vi "Calculate_(11)_Local_Cost_F()-1.vi"(4 "[IN] Dot matrix with statuses \nfor potentially moving dots":i16[][](array[numeric]), 5 "[IN] Still connected\ntracks in group":T1, 6 "[IN] Potentially\nMoving (X,Y)":dbl[][](array[numeric]), 7 "[IN] Subtracks":T2(array[cluster]), 8 "error IN":errorcluster, 9 "[IN] Areas particles\nPrimary Detected":dbl[][](array[numeric]), 10 "[IN] Primary \n(X,Y) Detected":dbl[][](array[numeric]), 11 "[IN] Cost function":i8[](array[numeric])) -> (0 "error OUT":errorcluster, 3 "[OUT] Cost function":i8[](array[numeric]))   [LabVIEW 2013]
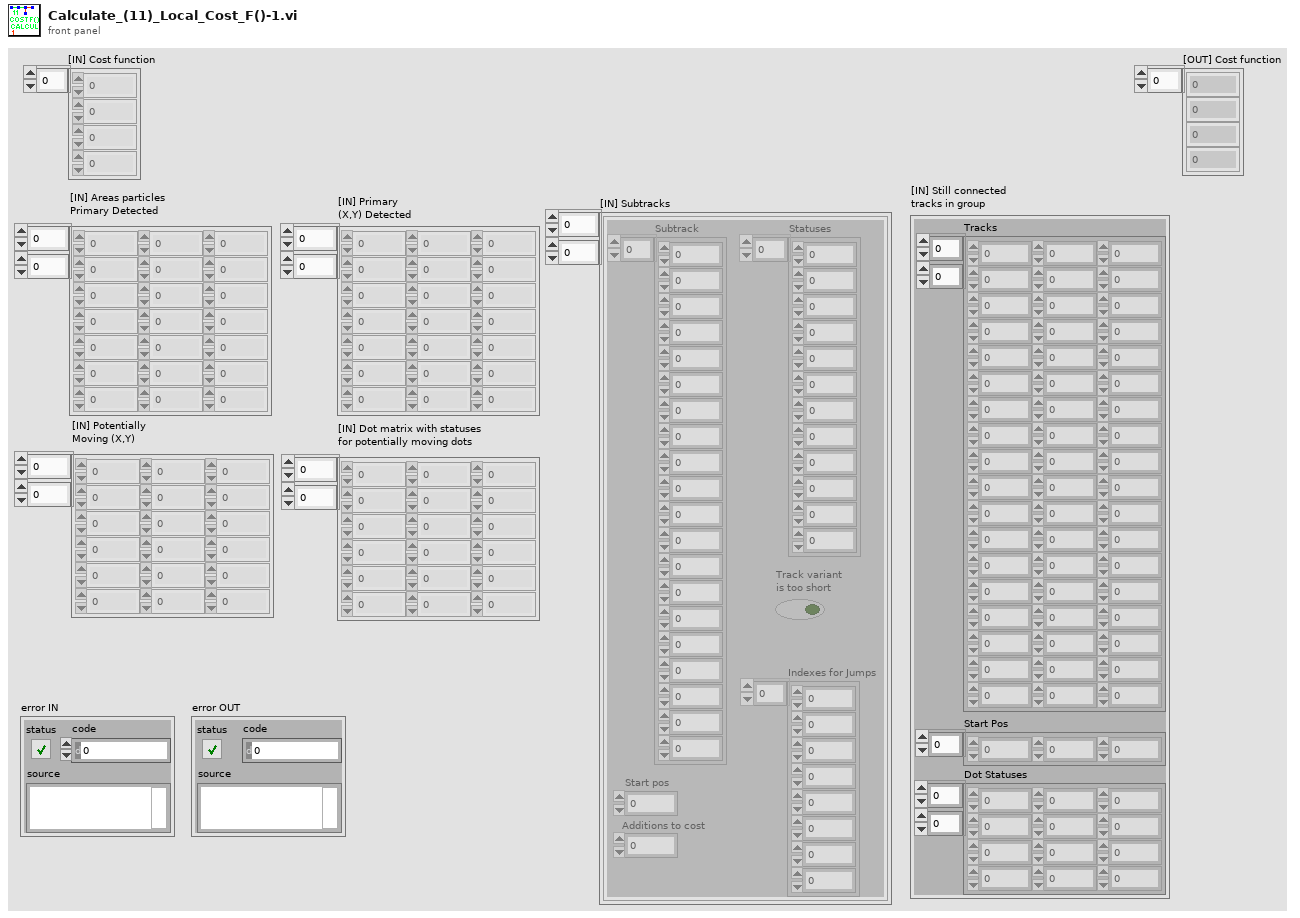
[diagram p1: front panel]
types:
  T1 = cluster{"Tracks":dbl[][], "Start Pos":i32[], "Dot Statuses":i16[][]}
  T2 = cluster{"Subtrack":dbl[], "Statuses":i16[], "Start pos":i32, "Additions to cost":i32, "Track variant \nis too short":bool, "Indexes for Jumps":i32[]}[][]
  T3 = cluster{"Subtrack":dbl[], "Statuses":i16[], "Start pos":i32, "Additions to cost":i32, "Track variant \nis too short":bool, "Indexes for Jumps":i32[]}[]
  T4 = cluster{"Subtrack":dbl[], "Statuses":i16[], "Start pos":i32, "Additions to cost":i32, "Track variant \nis too short":bool, "Indexes for Jumps":i32[]}
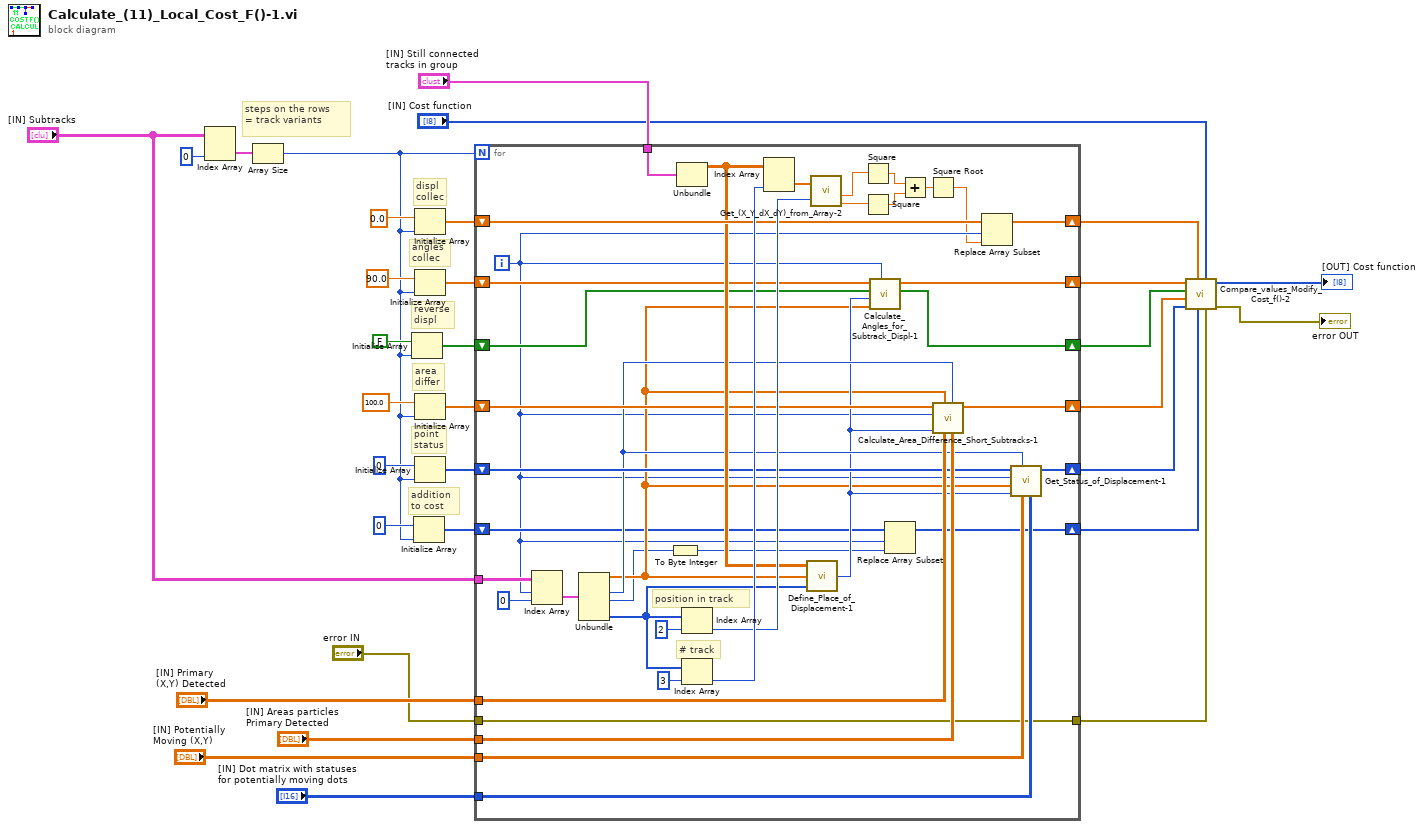
[diagram p0: block diagram]
diagram:
  # "steps on the rows\n= track variants"
  # "addition \nto cost"
  # "point\nstatus"
  # "area \ndiffer"
  # "reverse \ndispl"
  # "angles \ncollec"
  # "displ \ncollec"
  n1 = Index Array(array="[IN] Subtracks", index (col)=0 ("disabled index (col)")) -> (element=w18:T3)  [unwired: 1 in]
  n2 = Array Size(array=w18) -> (size(s)=w17:i32)
  n3 = Initialize Array(FALSE, w17) -> (w27:bool[])
  n4 = Initialize Array(i8 0, w17) -> (w21:i8[])
  n5 = Initialize Array(0.0, w17) -> (w31:dbl[])
  n6 = Initialize Array(90.0, w17) -> (w29:dbl[])
  n7 = Initialize Array(100.0, w17) -> (w25:dbl[])
  n8 = Initialize Array(i16 0, w17) -> (w23:i16[])
  n9 = for {
    N: w17 -> [_]
    tunnel: "[IN] Subtracks" -> [w72]
    tunnel: "[IN] Still connected\ntracks in group" -> [w67]
    shift-right: [w62] -> w6
    shift-left: w31 -> [w63]
    shift-right: [w58] -> w10
    shift-left: w29 -> [w59]
    shift-right: [w56] -> w9
    shift-left: w27 -> [w57]
    tunnel: "[IN] Primary \n(X,Y) Detected" -> [w52]
    tunnel: "[IN] Areas particles\nPrimary Detected" -> [w54]
    shift-right: [w53] -> w8
    shift-left: w25 -> [w55]
    tunnel: "[IN] Potentially\nMoving (X,Y)" -> [w47]
    tunnel: "[IN] Dot matrix with statuses \nfor potentially moving dots" -> [w46]
    shift-right: [w45] -> w7
    shift-left: w23 -> [w51]
    shift-right: [w40] -> w4
    shift-left: w21 -> [w44]
    tunnel: "error IN" -> [w33]
    tunnel: [w33] -> w2
    i -> [w43]
    # "# track"
    # "position in track"
    n10 = Index Array(array=w72, index (row)=w43, index (col)=0 ("disabled index (col)")) -> (element=w70:T4)
    n11 = Unbundle(w70) -> ("Subtrack"=w48:dbl[], "Start pos"=w50:i32, "Additions to cost"=w42:i32, "Indexes for Jumps"=w60:i32[])  [unwired: 2 out]
    n12 = To Byte Integer(number=w42) -> (8bit integer=w41:i8)
    n13 = Unbundle(w67) -> ("Tracks"=w61:dbl[][])  [unwired: 2 out]
    n14 = Index Array(array=w60, index=2) -> (element=w64:i32)
    n15 = Index Array(array=w60, index=3) -> (element=w66:i32)
    n16 = Index Array(array=w61, index (col)=w66) -> (element=w65:dbl[])  [unwired: 1 in]
    n17 = call "Define_Place_of_Displacement-1.vi"("[IN] Indexes for Jumps"=w60, "[IN] Subtrack"=w48, "[IN] Tracks"=w61) -> ("[OUT] Index of \"11\" Dis\nplacement in Subtrack"=w49:i32)  [unwired: 2 in]
    n18 = call "Get_(X_Y_dX_dY)_from_Array-2.vi"("(X,Y,dX,dY)"=w65, "Index of Displacement"=w64) -> ("dX"=w36:dbl, "dY"=w35:dbl)  [unwired: 2 out]
    n19 = Square(x=w36) -> (x^2=w39:dbl)
    n20 = Square(x=w35) -> (x^2=w38:dbl)
    n21 = call "Calculate_Angles_for_Subtrack_Displ-1.vi"("[IN] Index of subtrack"=w43, "[IN] Subtrack"=w48, "[IN] Index of \"11\" Dis-\nplacement in Subtrack"=w49, "[IN] Reverse Displ or Not"=w57, "[IN] Array with Angles \nBetween Displacement"=w59) -> ("[OUT] Reverse displacement or not"=w56:bool[], "[OUT] Angles betwe\nen two displacements"=w58:dbl[])  [unwired: 3 in]
    n22 = Replace Array Subset(array=w44, new element=w41, index=w43) -> (w40:i8[])
    n23 = Add(x=w39, y=w38) -> (x+y=w37:dbl)
    n24 = Square Root(x=w37) -> (sqrt(x)=w34:dbl)
    n25 = call "Calculate_Area_Difference_Short_Subtracks-1.vi"("[IN] Areas particles\nPrimary Detected"=w54, "[IN] Start pos"=w50, "[IN] Primary \n(X,Y) Detected"=w52, "[IN] Subtrack"=w48, "[IN] Index of \"11\" Dis-\nplacement in Subtrack"=w49, "[IN] Index of\n subtrack"=w43, "[IN] Areas \ndifference"=w55) -> ("[OUT] Areas \ndifference"=w53:dbl[])  [unwired: 4 in]
    n26 = Replace Array Subset(array=w63, new element=w34, index=w43) -> (w62:dbl[])
    n27 = call "Get_Status_of_Displacement-1.vi"("[IN] Dot matrix with statuses\nfor potentially moving dots"=w46, "[IN] Potentially\nMoving (X,Y)"=w47, "[IN] Start pos"=w50, "[IN] Index of Problem\nPoint in Subtrack"=w49, "[IN] Subtrack"=w48, "[IN] Index of\n subtrack"=w43, "[IN] Displace-\nment Statuses"=w51) -> ("[OUT] Displace\nment Statuses"=w45:i16[])  [unwired: 4 in]
  }
  n28 = call "Compare_values_Modify_Cost_f()-2.vi"("error IN"=w2, "[IN] Cost function"="[IN] Cost function", "[IN] Additions to cost"=w4, "[IN] Array of displa\ncement differences"=w6, "[IN] Statuses of points"=w7, "[IN] Areas \ndifferences"=w8, "[IN] Reverse or not"=w9, "[IN] Angles betwe\nen displacements"=w10) -> ("error OUT"=→"error OUT":errorcluster, "[OUT] Cost function"=→"[OUT] Cost function":i8[])  [unwired: 2 in]
